vi "DrawToPictureCore.vi"(5 "Pixel Formats":T1, 7 "Top Left Point":T2, 8 "error in (no error)":errorcluster, 11 "Buffer In":refnum<class "Buffer.lvclass">) -> (0 "error out":errorcluster, 3 "Picture":picture)   [LabVIEW 2020, in "Buffer.lvclass"]
uses:
  Buffer.lvclass
  Buffer.lvclass/Buffer.ctl
  bin/gindustrialcam_32-1.dll
  Picture Top Left Point Offset.ctl
  Pixel Formats.ctl
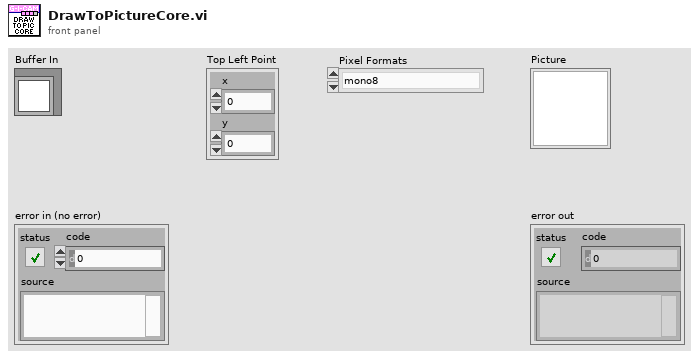
[diagram p1: front panel]
types:
  T1 = typedef "Buffer.lvclass/Pixel Formats.ctl" = enum16{"mono8", "mono10", "mono10p", "mono12", "mono12p", "mono14", "mono14p", "mono16", "RGB8", "BGR8"}
  T2 = typedef "Buffer.lvclass/Picture Top Left Point Offset.ctl" = cluster{"x":i16, "y":i16}
  T3 = cluster{"op_code":i16, "length":i32, "image_bytes_length":i32, "top":i16, "left":i16, "bottom":i16, "right":i16, "bitwidth":i16, "foreground":u32, "background":u32}
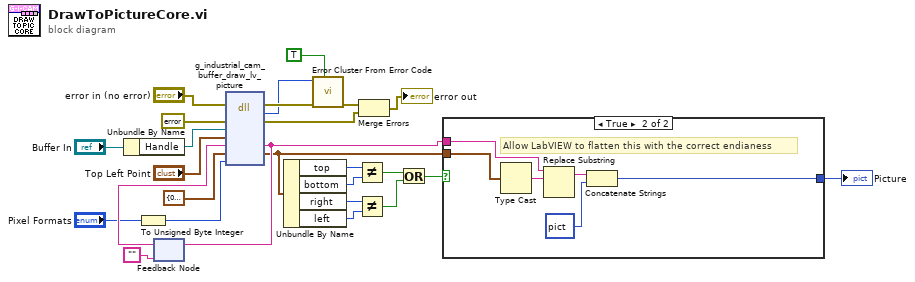
[diagram p0: block diagram]
diagram:
  n1 = Unbundle By Name("Buffer In") -> ("Handle"=w1:refnum<data-value>)
  n2 = To Unsigned Byte Integer(number="Pixel Formats") -> (unsigned 8bit integer=w2:u8)
  n3 = feedback #1("" ("Empty String Constant")) -> (w14:string)
  n4 = dll-call lib="C:/serenial/lib/g-industrial-camera/LabVIEW/g_industrial_cam/bin/gindustrialcam_*-1.*" fn="g_industrial_cam_buffer_draw_lv_picture" ("g_ar_toolkit.*.*:g_ar_tk_image_draw_picture")(error in="error in (no error)", "error_cluster"=errorcluster {"status"=FALSE, "code"=0, "source"=""} ("error constant"), "EDVR src"=w1, "top_left"="Top Left Point", "picture"=w14, "op_header"=T3 {"op_code"=0, "length"=0, "image_bytes_length"=0, "top"=0, "left"=0, "bottom"=0, "right"=0, "bitwidth"=0, "foreground"=0, "background"=0}, "pixel_format"=w2) -> (error out=w18:errorcluster, "return type"=w17:i32, "error_cluster"=w16:errorcluster, "picture"=w15:string, "op_header"=w11:T3)  [unwired: 5 in, 1 out]
  n5 = feedback-in #1(w15) -> ()
  n6 = Unbundle By Name(w11) -> ("top"=w10:i16, "bottom"=w9:i16, "right"=w7:i16, "left"=w6:i16)
  n7 = call <vilib>:"Error Cluster From Error Code.vi"("show call chain? (False)"=TRUE, "error in (no error)"=w18, "error code (0)"=w17) -> ("error out"=w25:errorcluster)  [unwired: 6 in]
  n8 = Not Equal?(x=w10, y=w9) -> (x != y?=w8:bool)
  n9 = Not Equal?(x=w7, y=w6) -> (x != y?=w4:bool)
  n10 = Merge Errors(w25, w16) -> (→"error out":errorcluster)
  n11 = Or(x=w8, y=w4) -> (x .or. y?=w5:bool)
  n12 = case shown="True" w5 {
    tunnel: [_ w30] -> w23
    tunnel: w11 -> [_ w29]
    tunnel: w15 -> [_ w28]
    frame False {
    }
    frame True {
      # "Allow LabVIEW to flatten this with the correct endianess"
      n13 = Type Cast(x=w29) -> (*(type *) &x=w32:string)  [unwired: 1 in]
      n14 = Replace Substring(4:w32, 5:w28) -> (1:w31:string)  [unwired: 2 in, 1 out]
      n15 = Concatenate Strings(w31, picture data[5B] ("empty picture")) -> (w30:picture)
    }
  }
  "Picture" <- w23
